vi "Read Variant DB.vi"(8 "error in (no error)":errorcluster, 11 "SeqGen Step Dictionary in":refnum<class "SeqGen Step Dictionary.lvclass">) -> (0 "error out":errorcluster, 2 "Variant DB":variant, 3 "SeqGen Step Dictionary out":refnum<class "SeqGen Step Dictionary.lvclass">)   [LabVIEW 2018, in "SeqGen Step Database.lvlib" / "SeqGen Step Dictionary.lvclass"]
uses:
  SeqGen Step Dictionary.lvclass
  SeqGen Step Dictionary.lvclass/SeqGen Step Dictionary.ctl
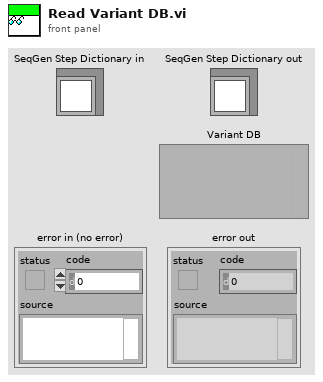
[diagram p1: front panel]
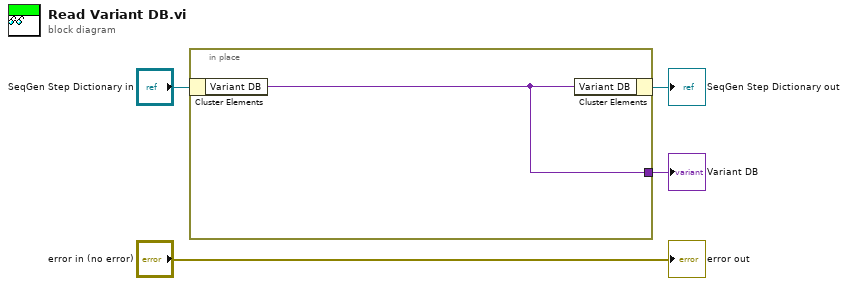
[diagram p0: block diagram]
diagram:
  n1 = in-place {
    in-place-border: [w5] -> w2
    n2 = in-place-cluster #1("SeqGen Step Dictionary in") -> ("Variant DB"=w5:variant)
    n3 = in-place-cluster #1("Variant DB"=w5) -> (→"SeqGen Step Dictionary out":refnum<class "SeqGen Step Dictionary.lvclass">)
  }
  "Variant DB" <- w2
  "error out" <- "error in (no error)"
